vi "Translation Stage Fine.vi"(8 "error in (no error)":errorcluster, 10 "Translation Stages.lvclass":refnum<class "Translation Stages.lvclass">, 11 "Translation Stage Fine In":refnum<class "Translation Stage Fine.lvclass">) -> (0 "error out":errorcluster, 3 "Translation Stage Fine Out":refnum<class "Translation Stage Fine.lvclass">)   [LabVIEW 2023, in "Translation Stage Fine.lvclass"]
uses:
  Translation Stage Fine.lvclass
  C:/LabVIEW-programs/Scanners/Scanner/Scanner.lvclass
  Instruments/Translation Stages/Translation Stages.lvclass
  C:/LabVIEW-programs/Instruments/Utility Classes/Scannable/Scannable.lvclass
  Scanner/Scanner.lvclass
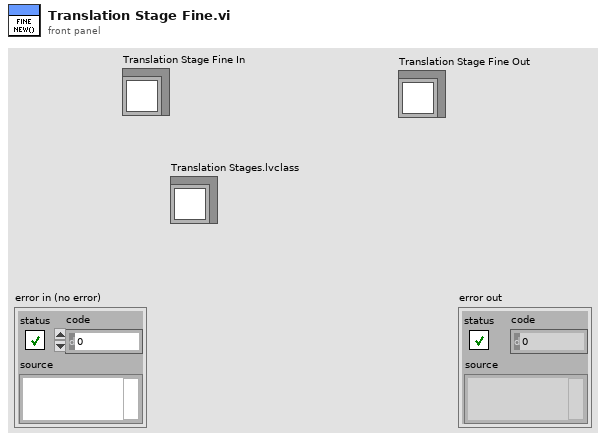
[diagram p1: front panel]
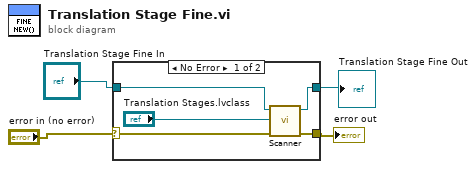
[diagram p0: block diagram]
diagram:
  n1 = case shown="No Error" "error in (no error)" {
    selector: "error in (no error)" -> [w7 w11]
    tunnel: [w6 w11] -> w1
    tunnel: [w9 w10] -> w3
    tunnel: "Translation Stage Fine In" -> [w8 w10]
    frame No Error {
      n2 = call "Scanner.vi"("error in (no error)"=w7, "Scannable"="Translation Stages.lvclass", "Scanner.lvclass in"=w8) -> ("error out"=w6:errorcluster, "Scanner.lvclass out"=w9:refnum<class "Translation Stage Fine.lvclass">)  [unwired: 1 in, 6 out]
    }
    frame Error {
    }
  }
  "Translation Stage Fine Out" <- w3
  "error out" <- w1
